vi "Send Tag Results to Inline.vi"(8 "Error in":errorcluster, 10 "Tag Results":dbl[](array[numeric]), 11 "Parameters":T1) -> (0 "Error out":errorcluster, 3 "Parameters dup":T1)   [LabVIEW 2014, in "Waveform-Processing-Custom-Device Engine.lvlib"]
uses:
  Waveform-Processing-Custom-Device Engine.lvlib
  Types/Async Parameters.ctl
  Types/Async FIFOs.ctl
  <vilib>/NI Veristand/Custom Device Waveform API/Single Waveform Read (DBL)/Single Waveform Read (DBL).lvclass
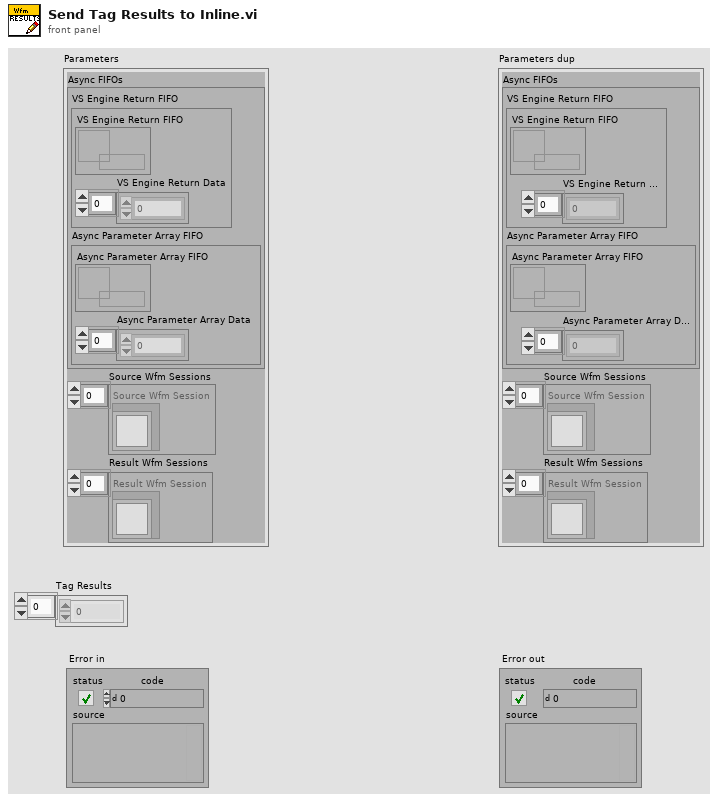
[diagram p1: front panel]
types:
  T1 = typedef "Waveform-Processing-Custom-Device Engine.lvlib/Async Parameters.ctl" = cluster{"Async FIFOs":T2, "Source Wfm Sessions":refnum<class "Single Waveform Read (DBL).lvclass">[], "Result Wfm Sessions":refnum<class "Single Waveform Read (DBL).lvclass">[]}
  T2 = typedef "Waveform-Processing-Custom-Device Engine.lvlib/Async FIFOs.ctl" = cluster{"VS Engine Return FIFO":cluster{"VS Engine Return FIFO":refnum<k33>, "VS Engine Return Data":dbl[]}, "Async Parameter Array FIFO":cluster{"Async Parameter Array FIFO":refnum<k33>, "Async Parameter Array Data":dbl[]}}
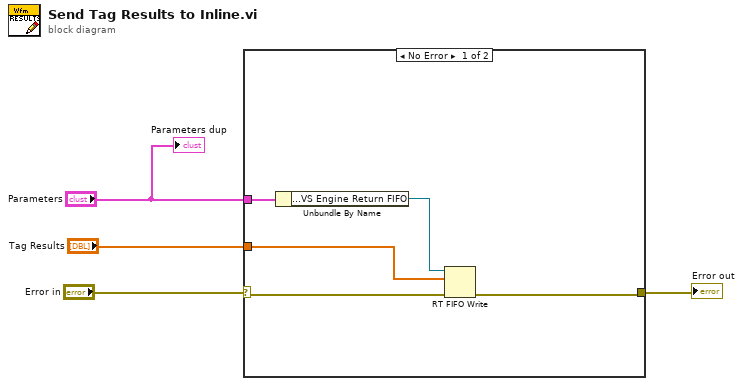
[diagram p0: block diagram]
diagram:
  n1 = case shown="No Error" "Error in" {
    selector: "Error in" -> [w8 w10]
    tunnel: [w7 w10] -> w3
    tunnel: "Parameters" -> [w9 _]
    tunnel: "Tag Results" -> [w5 _]
    frame No Error {
      n2 = Unbundle By Name(w9) -> ("Async FIFOs.VS Engine Return FIFO.VS Engine Return FIFO"=w6:refnum<k33>)
      n3 = RT FIFO Write(0:w6, 1:w5, 3:w8) -> (11:w7:errorcluster)  [unwired: 2 in, 3 out]
    }
    frame Error {
    }
  }
  "Error out" <- w3
  "Parameters dup" <- "Parameters"
